vi "test Basic Splitting of Elements - Package Only.vi"(8 "error in (no error)":errorcluster, 11 "TestCase in":refnum<class "Package List Tests.lvclass">) -> (0 "error out":errorcluster, 3 "TestCase out":refnum<class "Package List Tests.lvclass">)   [LabVIEW 2015, in "Package List Tests.lvclass"]
uses:
  Package List Tests.lvclass
  <vilib>/addons/_JKI Toolkits/VI Tester/TestCase.llb/TestCase.lvclass
  G CLI VIP.lvlib
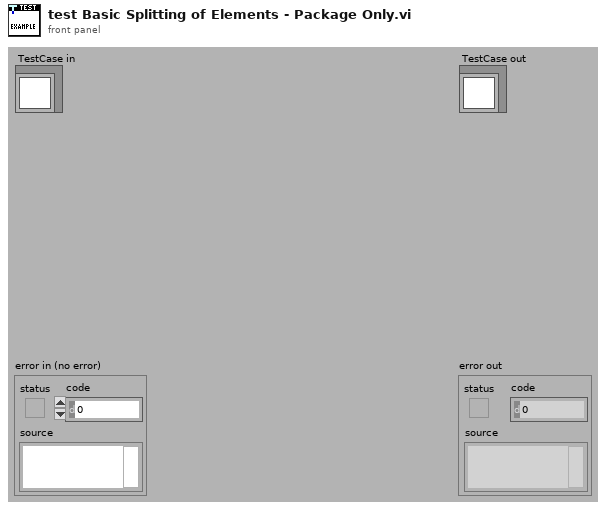
[diagram p1: front panel]
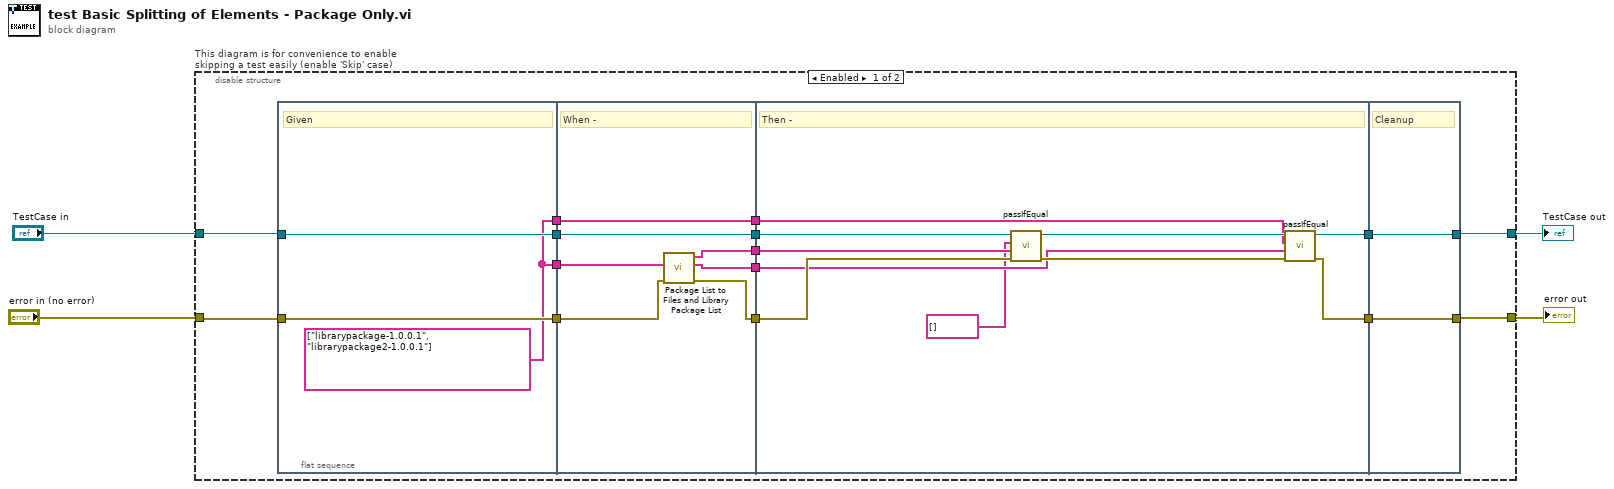
[diagram p0: block diagram]
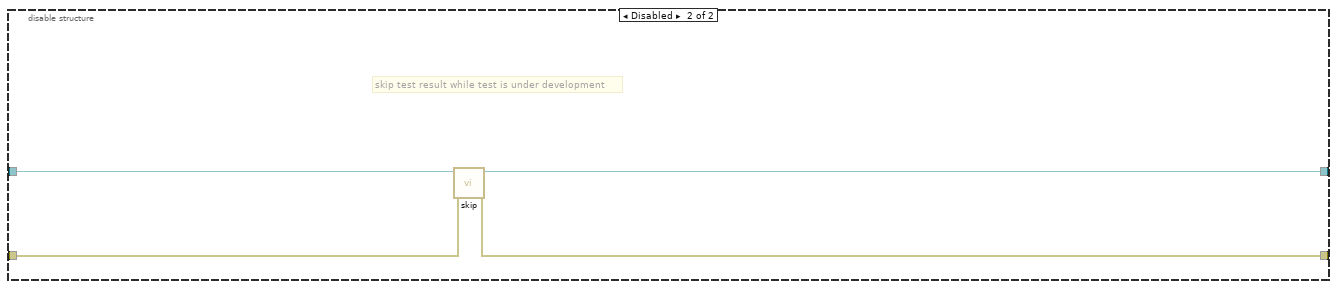
[diagram p2: hidden frame]
diagram:
  n1 = disable-structure "This diagram is for convenience to enable skipping a test easily (enable 'Skip' case)" shown="Enabled" {
    disable-tunnel: "TestCase in" -> [w14 w45]
    disable-tunnel: [w12 w43] -> w1
    disable-tunnel: [w11 w44] -> w3
    disable-tunnel: "error in (no error)" -> [w13 w42]
    frame Enabled {
      n2 = flat-sequence {
        tunnel: w13 -> [w21]
        tunnel: w14 -> [w22]
        tunnel: [w22] -> w19
        tunnel: [w21] -> w18
        tunnel: [w20] -> w10
        tunnel: [w20] -> w5
        tunnel: [w29] -> w17
        tunnel: w19 -> [w29]
        tunnel: w18 -> [w25]
        tunnel: w10 -> [w28]
        tunnel: [w27] -> w9
        tunnel: [w26] -> w8
        tunnel: [w24] -> w7
        tunnel: [w23] -> w6
        tunnel: w5 -> [w23]
        tunnel: [w34] -> w16
        tunnel: [w35] -> w15
        tunnel: w17 -> [w39]
        tunnel: w9 -> [w33]
        tunnel: w8 -> [w32]
        tunnel: w7 -> [w38]
        tunnel: w6 -> [w30]
        tunnel: [w41] -> w11
        tunnel: [w40] -> w12
        tunnel: w16 -> [w40]
        tunnel: w15 -> [w41]
        frame #0 {
          w20 = string[] ["librarypackage-1.0.0.1", "librarypackage2-1.0.0.1"]
          # "Given"
        }
        frame #1 {
          # "When -"
          n3 = call "Package List to Files and Library Package List.vi"("error in (no error)"=w25, "Packages"=w28) -> ("error out"=w24:errorcluster, "Library Packages"=w26:string[], "File Packages"=w27:string[])  [unwired: 7 in]
        }
        frame #2 {
          # "Then -"
          n4 = call-dynamic "passIfEqual.vi"("error in (no error)"=w38, "y"=w33, "x"=string[] [], "TestCase in"=w39) -> ("error out"=w36:errorcluster, "TestCase out"=w37:refnum<class "Package List Tests.lvclass">)  [unwired: 6 in]
          n5 = call-dynamic "passIfEqual.vi"("error in (no error)"=w36, "y"=w32, "x"=w30, "TestCase in"=w37) -> ("error out"=w35:errorcluster, "TestCase out"=w34:refnum<class "Package List Tests.lvclass">)  [unwired: 6 in]
        }
        frame #3 {
          # "Cleanup"
        }
      }
    }
    frame Disabled {
      # "skip test result while test is under development"
      n6 = call <vilib>:"skip.vi"("error in (no error)"=w42, "TestCase in"=w45) -> ("error out"=w44:errorcluster, "TestCase out"=w43:refnum<class "Package List Tests.lvclass">)  [unwired: 8 in]
    }
  }
  "error out" <- w3
  "TestCase out" <- w1
